vi "CI_IMAQ_SettingsEditor.vi"(11 "Camera state":variant) -> (3 "Camera state (out)":variant)   [LabVIEW 2011]
uses:
  GenericIMAQCameraInstance.ctl
  Main/Camera/GenericCameraConfigType.ctl
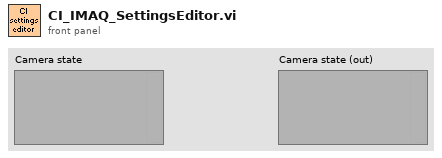
[diagram p1: front panel]
types:
  T1 = typedef "GenericIMAQCameraInstance.ctl" = cluster{"Session":refnum<k11>, "Settings":T2}
  T2 = typedef "GenericCameraConfigType.ctl" = cluster{"Framerate (Hz)":i32, "Exposure time (us)":i32, "Image size":cluster{"Width":i32, "Height":i32}, "Number of buffers":i32}
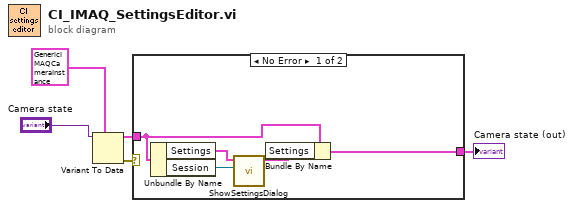
[diagram p0: block diagram]
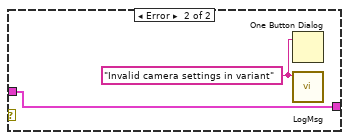
[diagram p2: hidden frame]
diagram:
  n1 = Variant To Data(type=T1 {"Session"=refnum, "Settings"={"Framerate (Hz)"=1, "Exposure time (us)"=50, "Image size"={"Width"=1280, "Height"=1024}, "Number of buffers"=0}} ("Camera data"), Variant="Camera state") -> (data=w4:T1, error out=w3:errorcluster)  [unwired: 1 in]
  n2 = case shown="No Error" w3 {
    tunnel: w4 -> [w8 w11]
    tunnel: [w9 w11] -> w2
    frame No Error {
      n3 = Unbundle By Name(w8) -> ("Settings"=w10:T2, "Session"=w6:refnum<k11>)
      n4 = call "ShowSettingsDialog.vi"("IMAQ Refnum in"=w6, "Camera (in)"=w10) -> ("Camera (out)"=w7:T2)  [unwired: 9 in]
      n5 = Bundle By Name(cluster=w8, "Settings"=w7) -> (w9:T1)
    }
    frame Error {
      w12 = "Invalid camera settings in variant" ("Invalid")
      n6 = One Button Dialog(message=w12) -> ()  [unwired: 1 in, 1 out]
      n7 = call "LogMsg.vi"("msg"=w12) -> ()  [unwired: 11 in]
    }
  }
  "Camera state (out)" <- w2
